vi "System Summary.vi"(1 "connection information":path, 2 "System Number":string) -> ()   [LabVIEW 2024]
uses:
  <vilib>/addons/database/Connection.llb/DB Tools Open Connec (Path).vi
  <vilib>/addons/database/_DB Variant To Data/Database Variant To Data.xnode
  <vilib>/addons/database/NI_Database_API.lvlib
panel:
  in  "OK":bool
  out "Rack":string
  out "Count":dbl
  out "ActivePositions":string
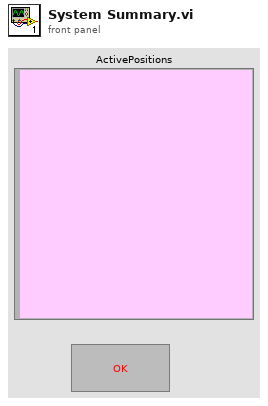
[diagram p1: front panel]
types:
  T1 = typedef "NI_Database_API.lvlib/Conn ObjectReference.ctl" = refnum<k1>
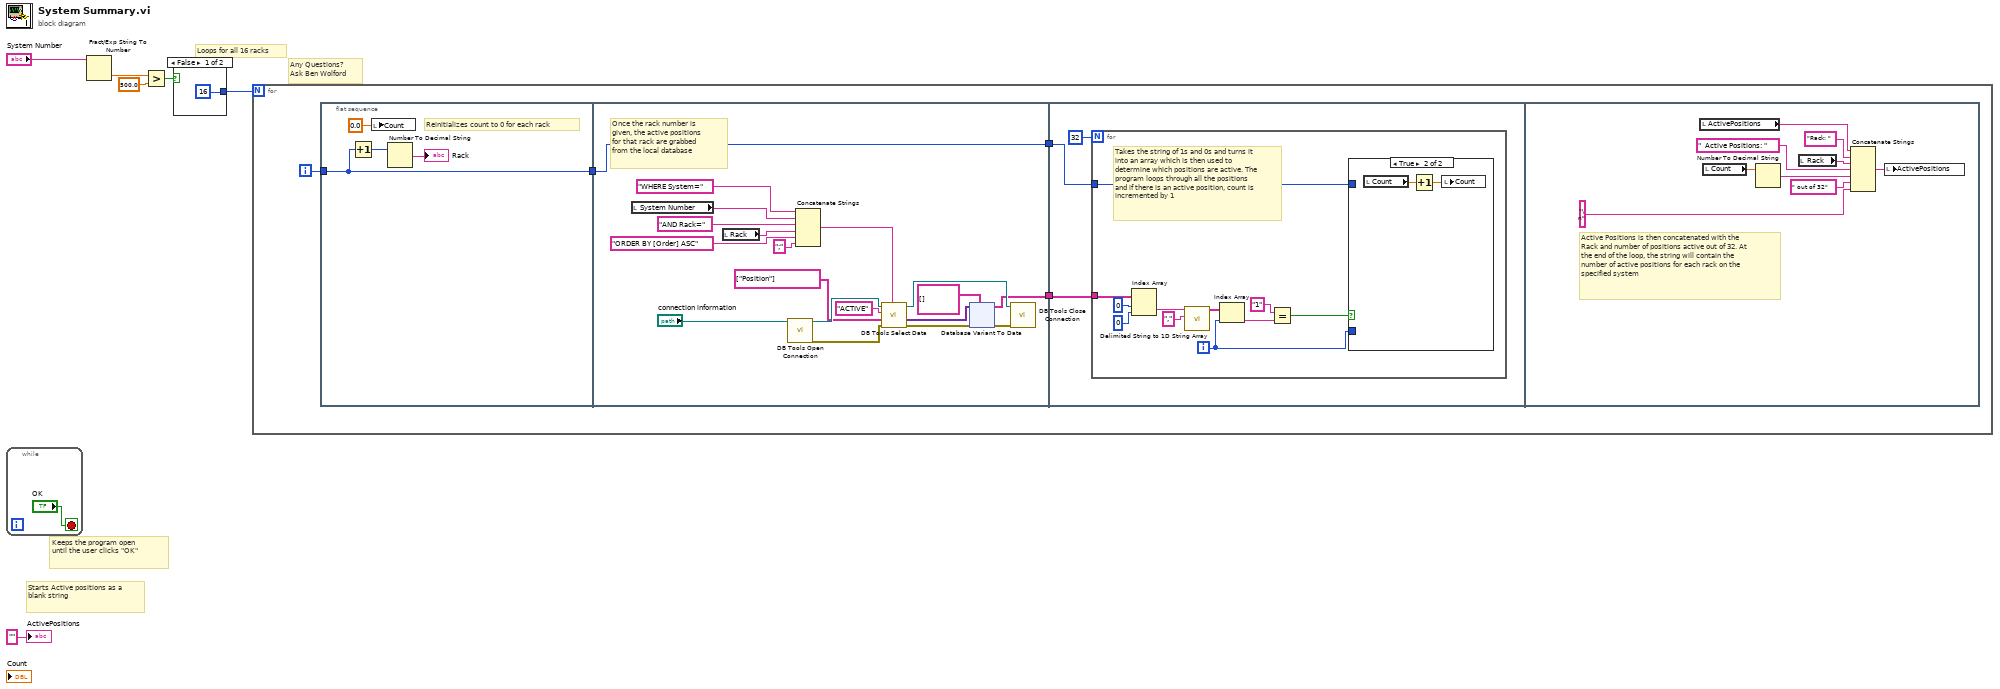
[diagram p0: block diagram]
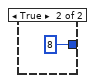
[diagram p2: hidden frame]
diagram:
  # "Starts Active positions as a blank string"
  # "Any Questions?\nAsk Ben Wolford"
  # "Keeps the program open until the user clicks \"OK\""
  # "Loops for all 16 racks"
  n1 = while {
    stop <- "OK" stop-if-true
  }
  n2 = Fract/Exp String To Number(string="System Number") -> (number=w3:dbl)  [unwired: 3 in, 1 out]
  n3 = Greater?(x=w3, y=500.0) -> (0:w1:bool)
  n4 = case shown="False" w1 {
    tunnel: [16 8] -> w5
    frame False {
    }
    frame True {
    }
  }
  n5 = for {
    N: w5 -> [_]
    i -> [w10]
    n6 = flat-sequence {
      tunnel: w10 -> [w14]
      tunnel: [w14] -> w11
      tunnel: [w36] -> w13
      tunnel: [w22] -> w12
      tunnel: w11 -> [w36]
      tunnel: w13 -> [w83]
      tunnel: w12 -> [w82]
      frame #0 {
        # "Reinitializes count to 0 for each rack"
        n7 = Increment(x=w14) -> (x+1=w15:i32)
        n8 = local write "Count"(0.0 ("Count")) -> ()
        n9 = Number To Decimal String(number=w15) -> (decimal integer string=→"Rack":string)  [unwired: 1 in]
      }
      frame #1 {
        # "Once the rack number is given, the active positions for that rack are grabbed from the local database"
        n10 = local read "System Number"() -> (w34:string)
        n11 = local read "Rack"() -> (w35:string)
        n12 = call-poly <vilib>:"DB Tools Open Connection.vi"("connection information"="connection information") -> ("error out"=w26:errorcluster, "connection reference"=w27:T1)  [unwired: 7 in]
        n13 = Concatenate Strings("WHERE System=" ("SQL Query"), w34, "AND Rack=", w35, "ORDER BY [Order] ASC" ("string"), ";" ("string")) -> (w21:string)
        n14 = call <vilib>:"DB Tools Select Data.vi"("condition"=w21, "error in (no error)"=w26, "columns"=string[] ["Position"], "table"="ACTIVE", "connection reference"=w27) -> ("error out"=w20:errorcluster, "data"=w24:variant[][], "connection reference out"=w28:T1)  [unwired: 1 in]
        n15 = xnode "Database Variant To Data"("database variant"=w24, "error in (no error)"=w20, "type"=string[][] [] ("table")) -> ("data"=w22:string[][], "error out"=w19:errorcluster)
        n16 = call <vilib>:"DB Tools Close Connection.vi"("error in (no error)"=w19, "connection reference"=w28) -> ()  [unwired: 5 in, 1 out]
      }
      frame #2 {
        n17 = for {
          N: 32 -> [_]
          tunnel: w83 -> [w94]
          tunnel: w82 -> [w92]
          i -> [w93]
          # "Takes the string of 1s and 0s and turns it into an array which is then used to determine which positions are active. The program loops through all the positions and if there is an active position, count is incremented by 1"
          n18 = Index Array(array=w92, index (row)=0 ("disabled index (row)"), index (col)=0 ("disabled index (col)")) -> (element=w91:string)
          n19 = call <vilib>:"Delimited String to 1D String Array.vi"("delimiter"=",", "delimited string"=w91) -> ("string array"=w90:string[])  [unwired: 9 in]
          n20 = Index Array(array=w90, index=w93) -> (element=w89:string)
          n21 = Equal?(x="1", y=w89) -> (x = y?=w84:bool)
          n22 = case shown="True" w84 {
            tunnel: w93 -> [_ _]
            tunnel: w94 -> [_ _]
            frame False {
            }
            frame True {
              n23 = local read "Count"() -> (w96:dbl)
              n24 = Increment(x=w96) -> (x+1=w95:dbl)
              n25 = local write "Count"(w95) -> ()
            }
          }
        }
      }
      frame #3 {
        # "Active Positions is then concatenated with the Rack and number of positions active out of 32. At the end of the loop, the string will contain the number of active positions for each rack on the specified system"
        n26 = local read "ActivePositions"() -> (w105:string)
        n27 = local read "Count"() -> (w103:dbl)
        n28 = Number To Decimal String(number=w103) -> (decimal integer string=w102:string)  [unwired: 1 in]
        n29 = local read "Rack"() -> (w104:string)
        n30 = Concatenate Strings(w105, "Rack: " ("string"), w104, "  Active Positions: " ("string"), w102, " out of 32" ("string"), "\n" ("string")) -> (w101:string)
        n31 = local write "ActivePositions"(w101) -> ()
      }
    }
  }
  "ActivePositions" <- "" ("ActivePositions")
